vi "is_moving.vi"(8 "error in":errorcluster, 11 "Newport Model 8742 in":refnum<class "Newport Model 8742.lvclass">) -> (0 "error out":errorcluster, 2 "Is moving?":bool, 3 "Newport Model 8742 out":refnum<class "Newport Model 8742.lvclass">)   [LabVIEW 2020, in "Newport Model 8742.lvclass"]
uses:
  Newport Model 8742.lvclass
  Newport Model 8742.lvclass/Newport Model 8742.ctl
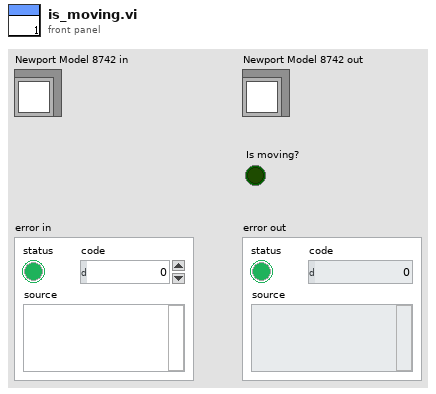
[diagram p1: front panel]
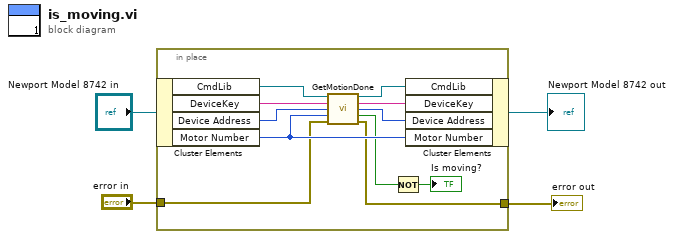
[diagram p0: block diagram]
diagram:
  n1 = in-place {
    in-place-border: "error in" -> [w8]
    in-place-border: [w5] -> w1
    n2 = in-place-cluster #1("Newport Model 8742 in") -> ("CmdLib"=w15:refnum<k24>, "DeviceKey"=w14:string, "Device Address"=w13:i32, "Motor Number"=w12:i32)
    n3 = call <instrlib>:"GetMotionDone.vi"("CmdLib In"=w15, "DeviceKey In"=w14, "Device Address In"=w13, "Motor"=w12, "error in (no error)"=w8) -> ("CmdLib Out"=w10:refnum<k24>, "DeviceKey Out"=w11:string, "Device Address Out"=w9:i32, "Is Motion Done"=w6:bool, "error out"=w5:errorcluster)  [unwired: 6 in]
    n4 = Not(x=w6) -> (.not. x?=→"Is moving?":bool)
    n5 = in-place-cluster #1("CmdLib"=w10, "DeviceKey"=w11, "Device Address"=w9, "Motor Number"=w12) -> (→"Newport Model 8742 out":refnum<class "Newport Model 8742.lvclass">)
  }
  "error out" <- w1
